vi "g_DI InputsALB.vi"(7 "Action":T3(ring), 9 "DIO in":bool, 10 "DI All in":T1, 11 "Parameter":T2) -> (2 "DI out":T1)   [LabVIEW 2017]
uses:
  CtrlRefs/DioDisplayALB.ctl
  CtrlRefs/DIO_ALB.ctl
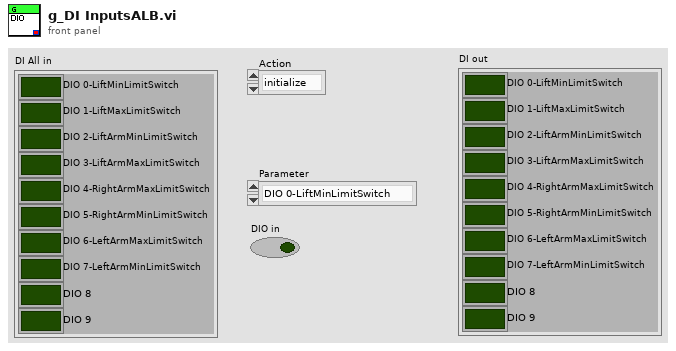
[diagram p1: front panel]
types:
  T1 = typedef "DioDisplayALB.ctl" = cluster{"DIO 0-LiftMinLimitSwitch":bool, "DIO 1-LiftMaxLimitSwitch":bool, "DIO 2-LiftArmMinLimitSwitch":bool, "DIO 3-LiftArmMaxLimitSwitch":bool, "DIO 4-RightArmMaxLimitSwitch":bool, "DIO 5-RightArmMinLimitSwitch":bool, "DIO 6-LeftArmMaxLimitSwitch":bool, "DIO 7-LeftArmMinLimitSwitch":bool, "DIO 8":bool, "DIO 9":bool}
  T2 = typedef "DIO_ALB.ctl" = enum16{"DIO 0-LiftMinLimitSwitch", "DIO 1-LiftMaxLimitSwitch", "DIO 2-LiftArmMinLimitSwitch", "DIO 3-LiftArmMaxLimitSwitch", "DIO 4-RightArmMaxLimitSwitch", "DIO 5-RightArmMinLimitSwitch", "DIO 6-LeftArmMaxLimitSwitch", "DIO 7-LeftArmMinLimitSwitch", "DIO 8-Unused", "DIO 9-Unused"}
  T3 = enum16{"initialize", "read", "write", "write all"}
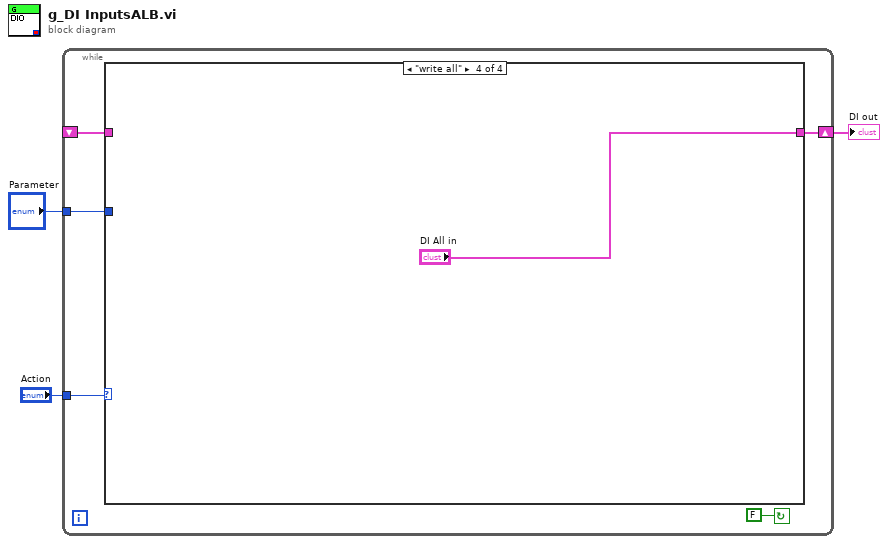
[diagram p0: block diagram]
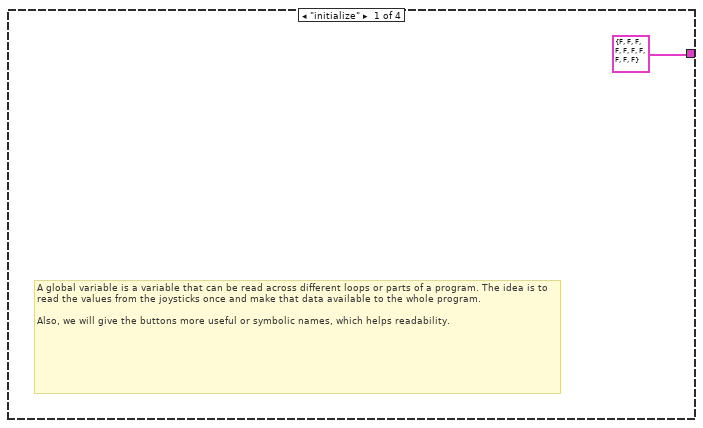
[diagram p2: hidden frame]
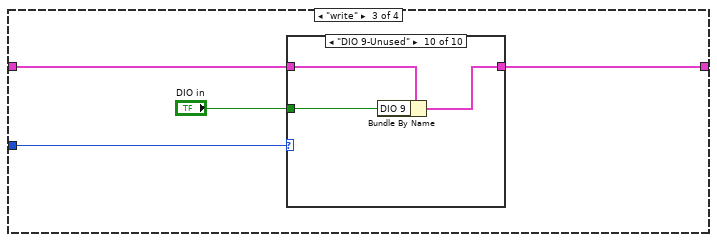
[diagram p4: hidden frame]
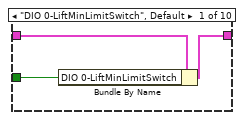
[diagram p5: hidden frame]
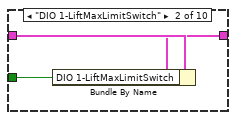
[diagram p6: hidden frame]
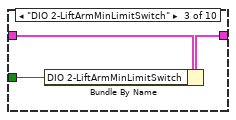
[diagram p7: hidden frame]
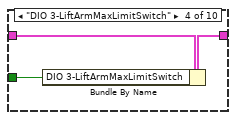
[diagram p8: hidden frame]
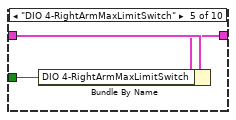
[diagram p9: hidden frame]
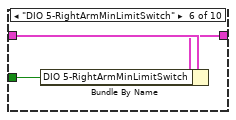
[diagram p10: hidden frame]
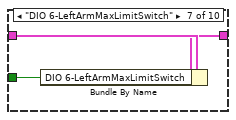
[diagram p11: hidden frame]
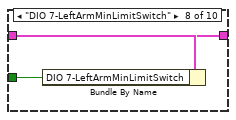
[diagram p12: hidden frame]
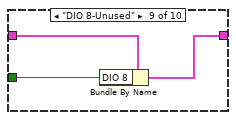
[diagram p13: hidden frame]
diagram:
  n1 = while {
    tunnel: "Action" -> [w7]
    shift-right: [w6] -> w1
    shift-left: _ -> [w5]
    tunnel: "Parameter" -> [w4]
    stop <- FALSE continue-if-true
    n2 = case shown="\"write all\"" w7 {
      tunnel: [T1 {"DIO 0-LiftMinLimitSwitch"=FALSE, "DIO 1-LiftMaxLimitSwitch"=FALSE, "DIO 2-LiftArmMinLimitSwitch"=FALSE, "DIO 3-LiftArmMaxLimitSwitch"=FALSE, "DIO 4-RightArmMaxLimitSwitch"=FALSE, "DIO 5-RightArmMinLimitSwitch"=FALSE, "DIO 6-LeftArmMaxLimitSwitch"=FALSE, "DIO 7-LeftArmMinLimitSwitch"=FALSE, "DIO 8"=FALSE, "DIO 9"=FALSE} ("DI out") w10 w13 "DI All in"] -> w6
      tunnel: w5 -> [_ w10 w14 _]
      tunnel: w4 -> [_ _ w12 _]
      frame "initialize" {
        # "A global variable is a variable that can be read across different loops or parts of a program. The idea is to read the values from the joysticks once and make that data available to the whole program.\n \nAlso, we will give the buttons more useful or symbolic names, which helps readability."
      }
      frame "read", Default {
      }
      frame "write" {
        n3 = case shown="\"DIO 9-Unused\"" w12 {
          tunnel: "DIO in" -> [w15 w18 w21 w24 w27 w30 w33 w36 w39 w42]
          tunnel: w14 -> [w17 w20 w23 w26 w29 w32 w35 w38 w41 w44]
          tunnel: [w16 w19 w22 w25 w28 w31 w34 w37 w40 w43] -> w13
          frame "DIO 0-LiftMinLimitSwitch", Default {
            n4 = Bundle By Name(cluster=w17, "DIO 0-LiftMinLimitSwitch"=w15) -> (w16:T1)
          }
          frame "DIO 1-LiftMaxLimitSwitch" {
            n5 = Bundle By Name(cluster=w20, "DIO 1-LiftMaxLimitSwitch"=w18) -> (w19:T1)
          }
          frame "DIO 2-LiftArmMinLimitSwitch" {
            n6 = Bundle By Name(cluster=w23, "DIO 2-LiftArmMinLimitSwitch"=w21) -> (w22:T1)
          }
          frame "DIO 3-LiftArmMaxLimitSwitch" {
            n7 = Bundle By Name(cluster=w26, "DIO 3-LiftArmMaxLimitSwitch"=w24) -> (w25:T1)
          }
          frame "DIO 4-RightArmMaxLimitSwitch" {
            n8 = Bundle By Name(cluster=w29, "DIO 4-RightArmMaxLimitSwitch"=w27) -> (w28:T1)
          }
          frame "DIO 5-RightArmMinLimitSwitch" {
            n9 = Bundle By Name(cluster=w32, "DIO 5-RightArmMinLimitSwitch"=w30) -> (w31:T1)
          }
          frame "DIO 6-LeftArmMaxLimitSwitch" {
            n10 = Bundle By Name(cluster=w35, "DIO 6-LeftArmMaxLimitSwitch"=w33) -> (w34:T1)
          }
          frame "DIO 7-LeftArmMinLimitSwitch" {
            n11 = Bundle By Name(cluster=w38, "DIO 7-LeftArmMinLimitSwitch"=w36) -> (w37:T1)
          }
          frame "DIO 8-Unused" {
            n12 = Bundle By Name(cluster=w41, "DIO 8"=w39) -> (w40:T1)
          }
          frame "DIO 9-Unused" {
            n13 = Bundle By Name(cluster=w44, "DIO 9"=w42) -> (w43:T1)
          }
        }
      }
      frame "write all" {
      }
    }
  }
  "DI out" <- w1
